vi "autoupdate.vi"() -> ()   [LabVIEW 2016, in "数据传输系统-02.lvlib"]
uses:
  update/update.lvlib
panel:
  out "结果字符串":string
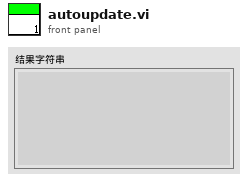
[diagram p1: front panel]
types:
  T1 = cluster{"主机":string, "用户":string, "密码":string, "远程路径":string, "下载文件名":string, "软件版本":string}
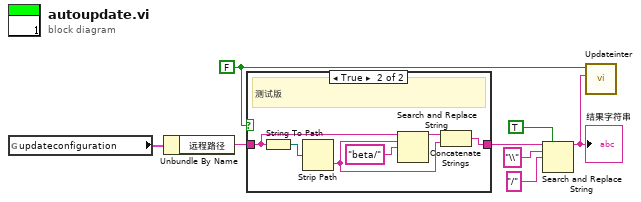
[diagram p0: block diagram]
diagram:
  w7 = FALSE ("测试版？")
  n1 = global read "断电保存全局.vi" "updateconfiguration"() -> (w8:T1)
  n2 = Unbundle By Name(w8) -> ("远程路径"=w6:string)
  n3 = case shown="True" w7 {
    tunnel: w6 -> [w9 w10]
    tunnel: [w9 w11] -> w4
    frame False {
      # "正式版"
    }
    frame True {
      # "测试版"
      n4 = String To Path(string=w10) -> (path=w12:path)
      n5 = Strip Path(path=w12) -> (name=w15:string)  [unwired: 1 out]
      n6 = Search and Replace String(input string=w10, search string=w15, replace string="beta/" ("字符串")) -> (result string=w14:string)  [unwired: 5 in, 3 out]
      n7 = Concatenate Strings(w14, w15) -> (w11:string)
    }
  }
  n8 = Search and Replace String(replace all?=TRUE ("替换全部？(F)"), input string=w4, search string="\\" ("替换字符串(\"\")"), replace string="/" ("分隔符(Tab)")) -> (result string=w1:string)  [unwired: 4 in, 3 out]
  "结果字符串" <- w1
  n9 = call "Updateinter.vi"("更新包远端地址"=w1, "测试版？"=w7) -> ()  [unwired: 10 in]
